vi "Read Spectrum Emission Mask Trace.vi"(0 "VISA resource name":refnum<visa-resource-name>, 5 "Trace Detection Mode (0:Positive Trace Data)":i32(ring) items=["Positive Trace Data", "Negative Trace Data"], 7 "Trace (0:REF)":i32(ring) items=["REF", "LOW1", "LOW2", "LOW3", "LOW4", "LOW5", "LOW6", "UPP1", "UPP2", "UPP3", "UPP4", "UPP5", "UPP6"], 11 "error in (no error)":errorcluster) -> (4 "VISA resource name out":refnum<visa-resource-name>, 6 "Spectrum Emission Mask Measurements":dbl[](array[numeric]), 15 "error out":errorcluster)   [LabVIEW 2020, in "Anritsu Signal Analyzer Series.lvlib"]
doc: "Reads SEM measurement Trace data"
uses:
  Anritsu Signal Analyzer Series.lvlib
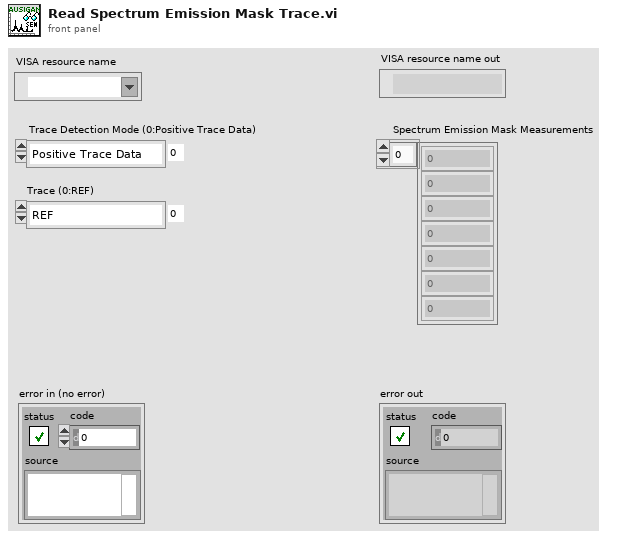
[diagram p1: front panel]
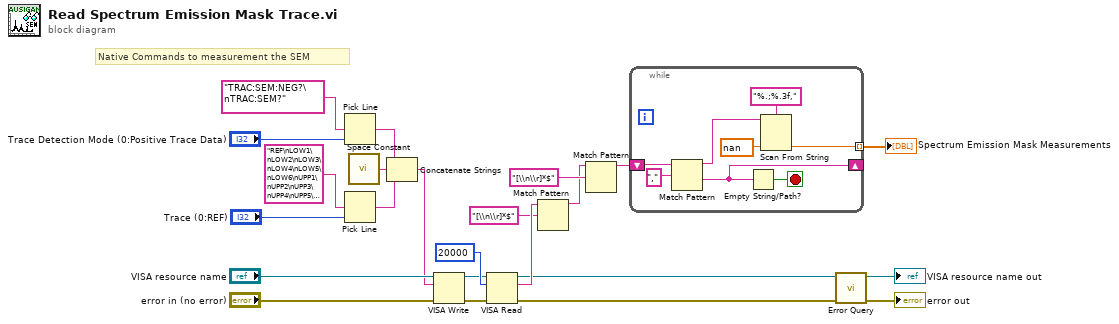
[diagram p0: block diagram]
diagram:
  # "Native Commands to measurement the SEM"
  n1 = Pick Line(multi-line string="TRAC:SEM:NEG?\nTRAC:SEM?" ("_CommandGet"), line index="Trace Detection Mode (0:Positive Trace Data)") -> (output string=w5:string)  [unwired: 1 in]
  n2 = Pick Line(multi-line string="REF\nLOW1\nLOW2\nLOW3\nLOW4\nLOW5\nLOW6\nUPP1\nUPP2\nUPP3\nUPP4\nUPP5\nUPP6" ("文字列"), line index="Trace (0:REF)") -> (output string=w1:string)  [unwired: 1 in]
  n3 = call <vilib>:"Space Constant.vi"() -> ("String"=w14:string)
  n4 = Concatenate Strings(w5, w14, w1) -> (w11:string)
  n5 = VISA Write(VISA resource name="VISA resource name", write buffer=w11, error in (no error)="error in (no error)") -> (VISA resource name out=w8:refnum<visa-resource-name>, error out=w9:errorcluster)  [unwired: 1 out]
  n6 = VISA Read(VISA resource name=w8, byte count=u32 20000 ("byte count (0)"), error in (no error)=w9) -> (VISA resource name out=w6:refnum<visa-resource-name>, read buffer=w13:string, error out=w7:errorcluster)  [unwired: 1 out]
  n7 = Match Pattern(string=w13, regular expression="[\\n\\r]*$") -> (before substring=w4:string)  [unwired: 1 in, 3 out]
  n8 = Match Pattern(string=w4, regular expression="[\\n\\r]*$") -> (before substring=w17:string)  [unwired: 1 in, 3 out]
  n9 = while {
    shift-right: [w24] -> _
    shift-left: w17 -> [w26]
    tunnel: [w30] -> w21 mode=indexing
    stop <- w29 stop-if-true
    n10 = Match Pattern(string=w26, regular expression=",") -> (before substring=w25:string, after substring=w24:string)  [unwired: 1 in, 2 out]
    n11 = Empty String/Path?(string/path=w24) -> (empty?=w29:bool)
    n12 = Scan From String(format string="%.;%.3f," ("Format String"), input string=w25, default 1=nan ("default value 1")) -> (output 1=w30:dbl)  [unwired: 2 in, 3 out]
  }
  "Spectrum Emission Mask Measurements" <- w21
  n13 = call "Error Query.vi"("error in (no error)"=w7, "VISA resource name"=w6) -> ("error out"=→"error out":errorcluster, "VISA resource name out"=→"VISA resource name out":refnum<visa-resource-name>)  [unwired: 6 in, 2 out]
